vi "Actor Core.vi"(8 "error in":errorcluster, 11 "Elevator Controller in":refnum<class "Sim Sensor Interface.lvclass">) -> (0 "error out":errorcluster, 3 "Actor out":refnum<class "Actor.lvclass">)   [LabVIEW 2019, in "Simulated Sensor Interface Actor.lvlib" / "Sim Sensor Interface.lvclass"]
doc: "(<B>Filename</B>: Actor Framework.lvlib:Actor.lvclass:Actor Core.vi)\n\nReceives messages to the actor, reacts to them, and initiates any error handling that may shut the actor down.\n\nDescendant classes may override this VI to append parallel tasks for the actor to complete while it handles messages. Overrides use the Call Parent Method node."
uses:
  Sim Sensor Interface.lvclass
  <vilib>/ActorFramework/Stop Msg/Stop Msg.lvclass
  <vilib>/ActorFramework/Actor/Actor.lvclass
  Sensor Interface/Sensor Interface/Sensor Interface.lvclass
  C:/Workspace/CLA/Elevator AF 2nd/Sensor Interface/Sensor Interface/Sensor Interface.lvclass
  C:/Program Files (x86)/National Instruments/LabVIEW 2019/vi.lib/ActorFramework/Actor/Actor.lvclass
  Elevator Controller/Elevator Controller Actor Messages/Set Enable Door Msg/Set Enable Door Msg.lvclass
panel:
  out "Elevator Position":u8(slide) scale=1.0..4.0
  # "[Covers: UI4] \n[Covers: UI4A]"
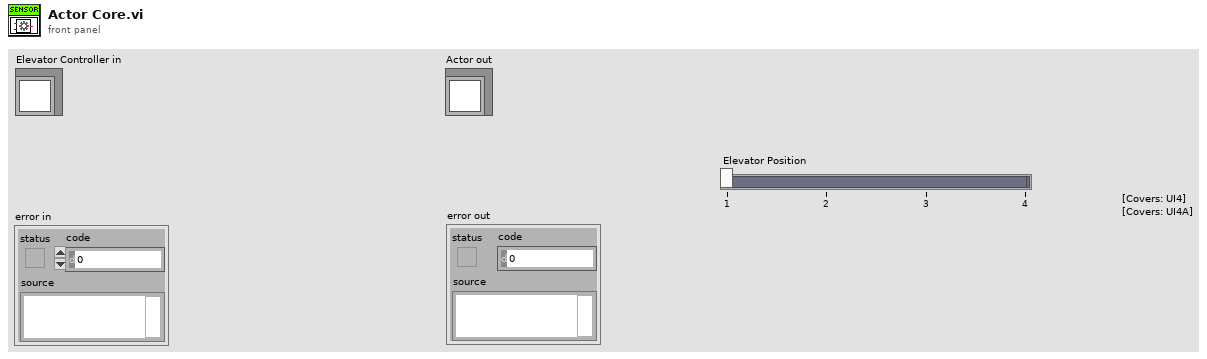
[diagram p1: front panel]
types:
  T1 = enum8{"Enabled", "Disabled", "Disabled and Grayed Out"}
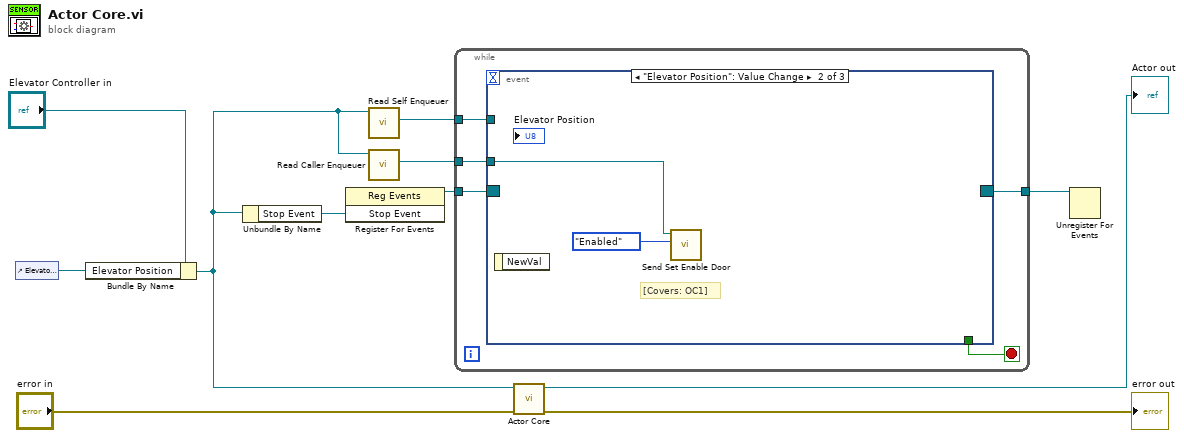
[diagram p0: block diagram]
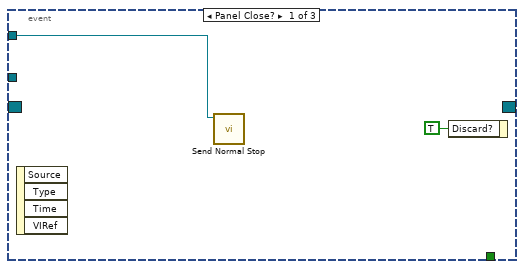
[diagram p2: hidden frame]
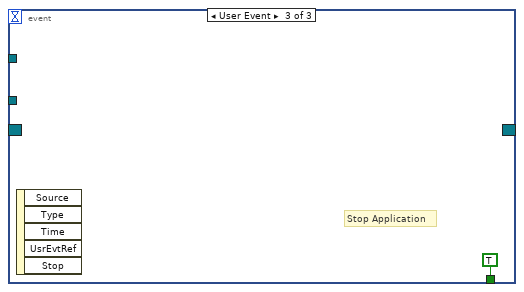
[diagram p3: hidden frame]
diagram:
  n1 = control-ref of="Elevator Position"() -> (w4:refnum<vi>)
  n2 = Bundle By Name(cluster="Elevator Controller in", "Elevator Position"=w4) -> (w2:refnum<class "Sim Sensor Interface.lvclass">)
  n3 = Unbundle By Name(w2) -> ("Stop Event"=w8:refnum<user-event>)
  n4 = register-events(w8) -> (reference out=w7:refnum<event-registration>)  [unwired: 2 in, 1 out]
  n5 = call <vilib>:"Read Self Enqueuer.vi"("Actor"=w2) -> ("Self Enqueuer"=w5:refnum<class "Message Enqueuer.lvclass">)  [unwired: 10 in]
  n6 = call <vilib>:"Read Caller Enqueuer.vi"("Actor"=w2) -> ("Caller Enqueuer"=w1:refnum<class "Message Enqueuer.lvclass">)  [unwired: 10 in]
  n7 = while {
    tunnel: w7 -> [w15]
    tunnel: [w14] -> w6
    tunnel: w5 -> [w13]
    tunnel: w1 -> [w12]
    stop <- w16 stop-if-true
    n8 = event shown="[1] \"Elevator Position\": Value Change" {
      selector: w15 -> [_ _ _]
      dyn-events: [_ _ _] -> w14
      timeout: _ -> [_ _ _]
      tunnel: [_ _ TRUE] -> w16
      tunnel: w13 -> [w17 _ _]
      tunnel: w12 -> [_ w20 _]
      event Panel Close? {
        n9 = event-data() -> ()  [unwired: 1 in, 4 out]
        n10 = call <vilib>:"Send Normal Stop.vi"("Message Enqueuer"=w17) -> ()  [unwired: 10 in, 1 out]
        n11 = event-data("Discard?"=TRUE) -> ()  [unwired: 1 in, 1 out]
      }
      event "Elevator Position": Value Change {
        # "[Covers: OC1]"
        n12 = event-data() -> ()  [unwired: 1 in, 1 out]
        n13 = call "Send Set Enable Door.vi"("Disabled"=T1."Enabled", "Message Enqueuer"=w20) -> ()  [unwired: 8 in, 2 out]
      }
      event User Event {
        # "Stop Application"
        n14 = event-data() -> ()  [unwired: 1 in, 5 out]
      }
    }
  }
  n15 = call-parent "Actor Core.vi"("error in"="error in", "Actor in"=w2) -> ("error out"=→"error out":errorcluster, "Actor out"=→"Actor out":refnum<class "Actor.lvclass">)  [unwired: 8 in]
  n16 = Unregister For Events(event registration refnum=w6) -> ()  [unwired: 1 in, 1 out]
